vi "PCO_Filter.vi"() -> (0 "PCO_Filter":T1, 1 "PCO_Filter_Raw":T2, 2 "Length":u16, 3 "Raw_Length":u16)   [LabVIEW 2020, in "Convert.lvlib"]
doc: "Use this template to build a VI to use as a subVI."
uses:
  Convert.lvlib
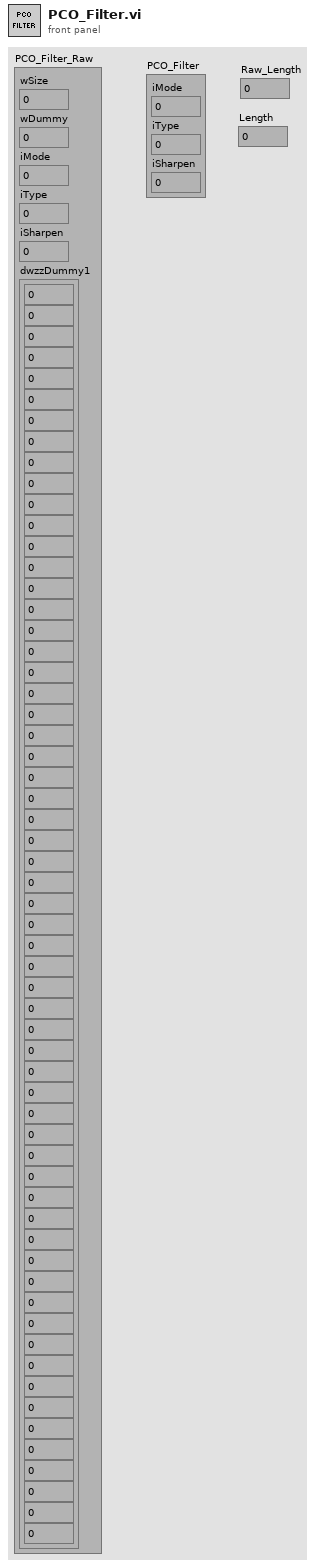
[diagram p1: front panel]
types:
  T1 = cluster{"iMode":i32, "iType":i32, "iSharpen":i32}
  T2 = cluster{"wSize":u16, "wDummy":u16, "iMode":i32, "iType":i32, "iSharpen":i32, "dwzzDummy1":cluster{u32, u32, u32, u32, u32, u32, u32, u32, u32, u32, u32, u32, u32, u32, u32, u32, u32, u32, u32, u32, u32, u32, u32, u32, u32, u32, u32, u32, u32, u32, u32, u32, u32, u32, u32, u32, u32, u32, u32, u32, u32, u32, u32, u32, u32, u32, u32, u32, u32, u32, u32, u32, u32, u32, u32, u32, u32, u32, u32, u32}}
  T3 = cluster{u32, u32, u32, u32, u32, u32, u32, u32, u32, u32, u32, u32, u32, u32, u32, u32, u32, u32, u32, u32, u32, u32, u32, u32, u32, u32, u32, u32, u32, u32, u32, u32, u32, u32, u32, u32, u32, u32, u32, u32, u32, u32, u32, u32, u32, u32, u32, u32, u32, u32, u32, u32, u32, u32, u32, u32, u32, u32, u32, u32}
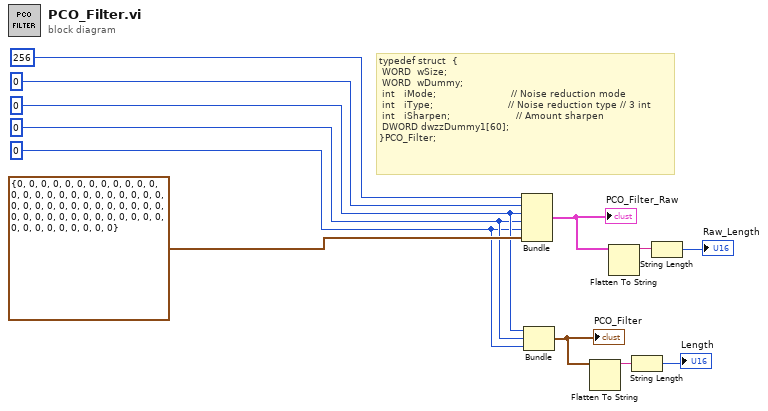
[diagram p0: block diagram]
diagram:
  w1 = 0 ("iSharpen")
  w2 = 0 ("iType")
  w3 = 0 ("iMode")
  # "typedef struct  {\n\tWORD  wSize;\n\tWORD  wDummy;\n\tint   iMode;                         // Noise reduction mode\n\tint   iType;                         // Noise reduction type // 3 int\n\tint   iSharpen;                      // Amount sharpen\n\tDWORD dwzzDummy1[60]; \n}PCO_Filter;"
  n1 = Bundle("wSize"=u16 256, "wDummy"=u16 0, "iMode"=w3, "iType"=w2, "iSharpen"=w1, "dwzzDummy1"=T3 {0, 0, 0, 0, 0, 0, 0, 0, 0, 0, 0, 0, 0, 0, 0, 0, 0, 0, 0, 0, 0, 0, 0, 0, 0, 0, 0, 0, 0, 0, 0, 0, 0, 0, 0, 0, 0, 0, 0, 0, 0, 0, 0, 0, 0, 0, 0, 0, 0, 0, 0, 0, 0, 0, 0, 0, 0, 0, 0, 0}) -> (w6:T2)  [unwired: 1 in]
  "PCO_Filter_Raw" <- w6
  n2 = Bundle("iMode"=w3, "iType"=w2, "iSharpen"=w1) -> (w12:T1)  [unwired: 1 in]
  "PCO_Filter" <- w12
  n3 = Flatten To String(anything=w12) -> (data string=w11:string)  [unwired: 3 in, 2 out]
  n4 = Flatten To String(anything=w6) -> (data string=w10:string)  [unwired: 3 in, 2 out]
  n5 = String Length(string=w11) -> (length=→"Length":i32)
  n6 = String Length(string=w10) -> (length=→"Raw_Length":i32)
